vi "Main.vi"(4 "출력 클러스터 2":T1, 5 "RowHdrs":string[](array[string]), 6 "Internal Control":string[][](table)=[["H01", "SYBR", "beta-Actin", "Unkn", "Fl1", "22.22", ""], ["H02", "SYBR", "beta-Actin", "Unkn", "Fl1", "22.27", ""], ["H03", "SYBR", "beta-Actin", "Unkn", "Fl2", "22.94", ""], ["H04", "SYBR", "beta-Actin", "Unkn", "Fl2", "22.82", ""], ["H05", "SYBR", "beta-Actin", "Unkn", "Fl3", "23.04", ""], ["H06", "SYBR", "beta-Actin", "Unkn", "Fl3", "22.72", ""], ["H07", "SYBR", "beta-Actin", "Unkn", "Pfl1", "22.09", ""], ["H08", "SYBR", "beta-Actin", "Unkn", "Pfl1", "22.09", ""], ["H09", "SYBR", "beta-Actin", "Unkn", "Pfl2", "21.57", ""], ["H10", "SYBR", "beta-Actin", "Unkn", "Pfl2", "21.16", ""], ["H11", "SYBR", "beta-Actin", "Unkn", "Pfl3", "21.80", ""], ["H12", "SYBR", "beta-Actin", "Unkn", "Pfl3", "21.93", ""]], 7 "Target Gene":string[][][](array[string])) -> (0 "Result":string[][](table), 1 "Plot data":cluster{i32[], dbl[]}[][](array[cluster]), 3 "Bar (or symbol) plot":picture[][](array[picture]))   [LabVIEW 2015]
uses:
  <vilib>/Analysis/baseanly.llb/Mean (DBL).vi
  <vilib>/Analysis/NI_AALBase.lvlib
panel:
  out "P-value":dbl[](array[numeric])
  out "Report format":string[][](table)
  out "Out":string[](array[string])
  out "Internal Control_Mean":string[](array[string])
  out "Internal Control_Data":string[](array[string])
  out "Gene List":string[](array[string])
  out "Target_Data":string[][](array[string])
  out "2^(-ddCt)":dbl[][](array[numeric])
  out "ddCt":dbl[][](array[numeric])
  out "AVG_dCt_Ctrl":dbl[](array[numeric])
  out "2^(-dCt)":dbl[][](array[numeric])
  out "dCt":dbl[][](array[numeric])
  out "Result Block":string[][][](array[string])
  out "RowHdrs":string[](array[string])
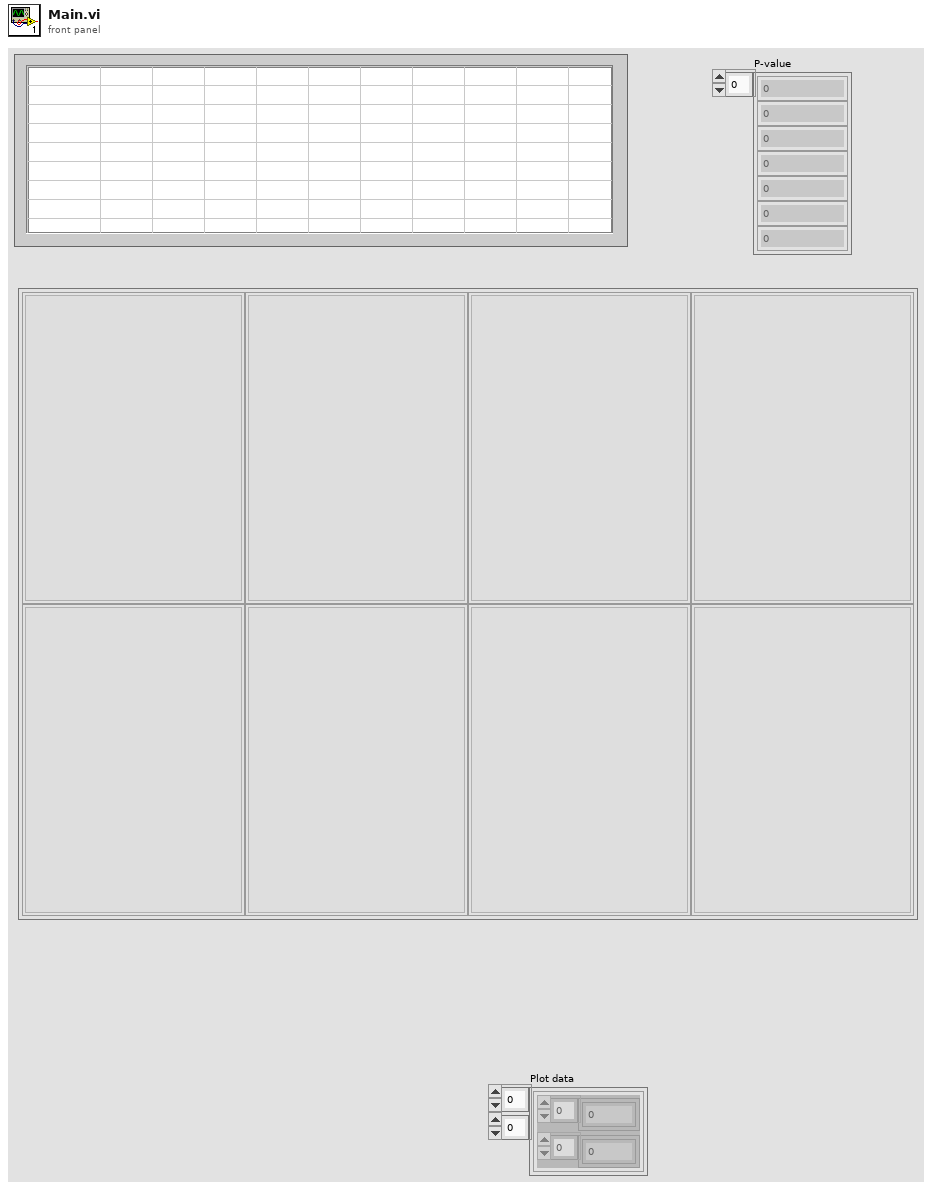
[diagram p1: front panel]
types:
  T1 = cluster{"Group #":dbl, "Biological replicate":dbl, "Technical replicate":dbl}
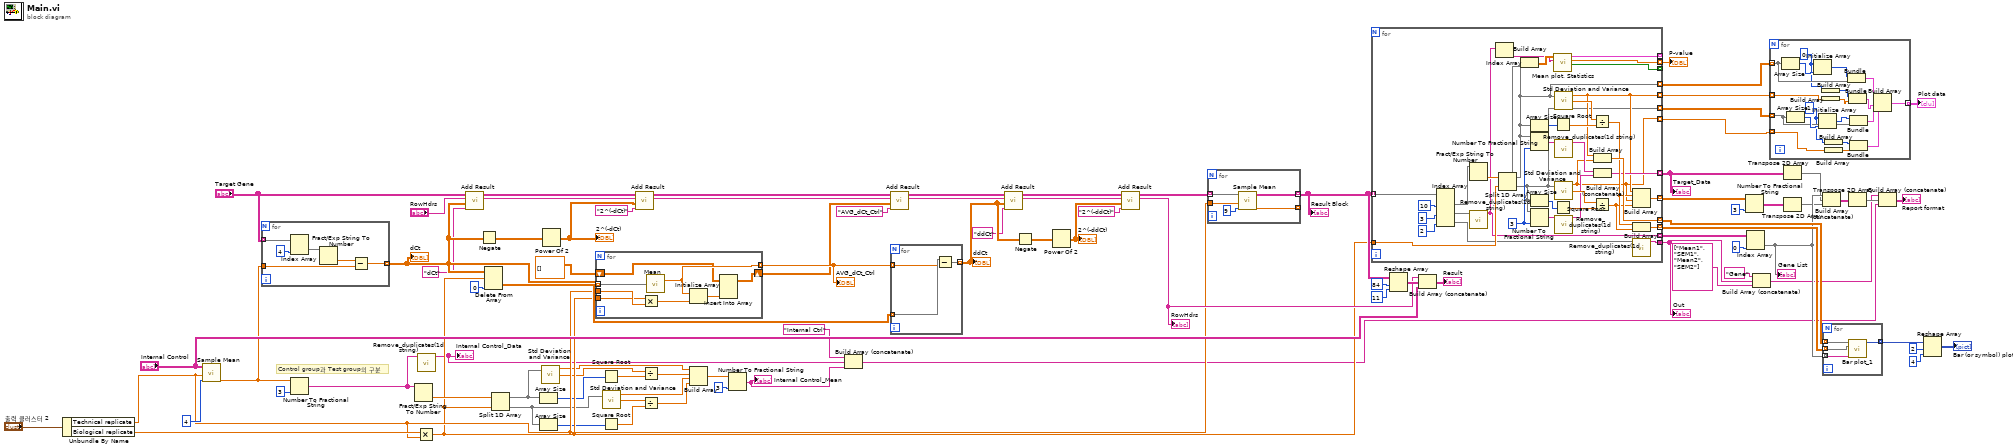
[diagram p0: block diagram]
diagram:
  # "Control group과 Test group의 구분"
  n1 = Unbundle By Name("출력 클러스터 2") -> ("Technical replicate"=w46:dbl, "Biological replicate"=w47:dbl)
  n2 = call "Sample Mean.vi"("Select Data"=4 ("비활성화된 인덱스 (열)"), "Technical replicate"=w46, "Input"="Internal Control") -> ("Sample Average"=w40:dbl[])  [unwired: 7 in, 1 out]
  n3 = for {
    tunnel: "Target Gene" -> [w95] mode=indexing
    tunnel: w40 -> [w91]
    tunnel: [w90] -> w81 mode=indexing
    n4 = Index Array(array=w95, index (col)=4 ("비활성화된 인덱스 (열)")) -> (element=w93:string[])  [unwired: 1 in]
    n5 = Fract/Exp String To Number(string=w93) -> (number=w92:dbl[])  [unwired: 3 in, 1 out]
    n6 = Subtract(x=w92, y=w91) -> (x-y=w90:dbl[])
  }
  "dCt" <- w81
  n7 = Number To Fractional String(number=w40, precision (6)=i16 3 ("정밀도(6)")) -> (F-format string=w38:string[])  [unwired: 2 in]
  n8 = Fract/Exp String To Number(string=w38) -> (number=w39:dbl[])  [unwired: 3 in, 1 out]
  n9 = call <userlib>:"Remove_duplicates(1d string).vi"("In"=w38) -> ("Out"=w9:string[])  [unwired: 10 in]
  "Internal Control_Data" <- w9
  n10 = Multiply(x=w47, y=w46) -> (x*y=w37:dbl)
  n11 = call "Add Result.vi"("Header"="dCt", "dCt"=w81, "RowHdrs Input"="RowHdrs", "Input"="Target Gene") -> ("RowHdrs Output"=w78:string[], "Output"=w79:string[][][])  [unwired: 6 in]
  n12 = Negate(x=w81) -> (-x=w89:dbl[][])
  n13 = Delete From Array(array=w81, length=w37, index (col)=0 ("비활성화된 인덱스 (열)")) -> (deleted portion=w87:dbl[][])  [unwired: 1 in, 1 out]
  n14 = Split 1D Array(array=w39, index=w37) -> (first subarray=w33:dbl[], second subarray=w29:dbl[])
  n15 = Array Size(array=w33) -> (size(s)=w34:i32)
  n16 = Array Size(array=w29) -> (size(s)=w32:i32)
  n17 = call <vilib>:"Std Deviation and Variance.vi"("X"=w33) -> ("mean"=w28:dbl, "standard deviation"=w35:dbl)  [unwired: 1 in, 1 out]
  n18 = Power Of 2(x=w89) -> (2^x=w77:dbl[][])
  "2^(-dCt)" <- w77
  n19 = for {
    tunnel: w87 -> [w103] mode=indexing
    tunnel: [w102] -> w86 mode=indexing
    shift-right: [w99] -> w59
    shift-left: dbl[][] [] -> [w101]
    tunnel: w37 -> [w97]
    tunnel: w46 -> [w98]
    n20 = Multiply(x=w97, y=w98) -> (x*y=w96:dbl)
    n21 = call-poly <vilib>:"Mean.vi"("X"=w103) -> ("mean"=w102:dbl)  [unwired: 1 out]
    n22 = Initialize Array(w102, w96) -> (w100:dbl[])
    n23 = Insert Into Array(array=w101, new element=w100) -> (w99:dbl[][])  [unwired: 2 in]
  }
  "AVG_dCt_Ctrl" <- w86
  n24 = Square Root(x=w34) -> (sqrt(x)=w36:dbl)
  n25 = Square Root(x=w32) -> (sqrt(x)=w30:dbl)
  n26 = call <vilib>:"Std Deviation and Variance.vi"("X"=w29) -> ("mean"=w26:dbl, "standard deviation"=w31:dbl)  [unwired: 1 in, 1 out]
  n27 = call "Add Result.vi"("Header"="2^(-dCt)", "dCt"=w77, "RowHdrs Input"=w78, "Input"=w79) -> ("RowHdrs Output"=w64:string[], "Output"=w63:string[][][])  [unwired: 6 in]
  n28 = Divide(x=w35, y=w36) -> (x/y=w27:dbl)
  n29 = Divide(x=w31, y=w30) -> (x/y=w25:dbl)
  n30 = Build Array(w28, w27, w26, w25) -> (w24:dbl[])
  n31 = Number To Fractional String(number=w24, precision (6)=i16 3 ("정밀도(6)")) -> (F-format string=w8:string[])  [unwired: 2 in]
  "Internal Control_Mean" <- w8
  n32 = Build Array (concatenate)("Internal Ctrl", w9, w8) -> (w7:string[])
  n33 = call "Add Result.vi"("Header"="AVG_dCt_Ctrl", "dCt"=w59, "RowHdrs Input"=w64, "Input"=w63) -> ("RowHdrs Output"=w61:string[], "Output"=w62:string[][][])  [unwired: 6 in]
  n34 = for {
    tunnel: w81 -> [w106] mode=indexing
    tunnel: w86 -> [w105] mode=indexing
    tunnel: [w104] -> w75 mode=indexing
    n35 = Subtract(x=w106, y=w105) -> (x-y=w104:dbl[])
  }
  "ddCt" <- w75
  n36 = call "Add Result.vi"("Header"="ddCt", "dCt"=w75, "RowHdrs Input"=w61, "Input"=w62) -> ("RowHdrs Output"=w73:string[], "Output"=w58:string[][][])  [unwired: 6 in]
  n37 = Negate(x=w75) -> (-x=w85:dbl[][])
  n38 = Power Of 2(x=w85) -> (2^x=w72:dbl[][])
  "2^(-ddCt)" <- w72
  n39 = call "Add Result.vi"("Header"="2^(-ddCt)", "dCt"=w72, "RowHdrs Input"=w73, "Input"=w58) -> ("RowHdrs Output"=w66:string[], "Output"=w57:string[][][])  [unwired: 6 in]
  "RowHdrs" <- w66
  n40 = for {
    tunnel: w57 -> [w111] mode=indexing
    tunnel: [w109] -> w56 mode=indexing
    tunnel: [w108] -> _ mode=indexing
    tunnel: w46 -> [w107]
    n41 = call "Sample Mean.vi"("Select Data"=9, "Technical replicate"=w107, "Input"=w111) -> ("Sample Average"=w108:dbl[], "Output"=w109:string[][])  [unwired: 7 in]
  }
  "Result Block" <- w56
  n42 = for {
    tunnel: w56 -> [w148] mode=indexing
    tunnel: [w138] -> w51 mode=indexing
    tunnel: [w137] -> w50 mode=indexing
    tunnel: w37 -> [w136]
    tunnel: [w133] -> w45 mode=indexing
    tunnel: [w128] -> w21 mode=indexing
    tunnel: [w120] -> w43 mode=indexing
    tunnel: [w122] -> w17
    tunnel: [w118] -> _ mode=indexing
    tunnel: [w117] -> w6 mode=indexing
    tunnel: [w116] -> _ mode=indexing
    tunnel: [w115] -> w5 mode=indexing
    tunnel: [w114] -> w3 mode=indexing
    tunnel: [w113] -> w4 mode=indexing
    tunnel: [w112] -> w2 mode=indexing
    w127 = i16 3 ("정밀도(6)")
    n43 = Index Array(array=w148, index (col) #1=10 ("비활성화된 인덱스 (열)"), index (col) #2=3 ("인덱스 (열)"), index (col) #3=2 ("인덱스 (열)")) -> (element #1=w146:string[], element #2=w125:string[], element #3=w123:string[])  [unwired: 3 in]
    n44 = Fract/Exp String To Number(string=w146) -> (number=w145:dbl[])  [unwired: 3 in, 1 out]
    n45 = call <userlib>:"Remove_duplicates(1d string).vi"("In"=w125) -> ("Out"=w120:string[])  [unwired: 10 in]
    n46 = Index Array(array=w120) -> (element=w119:string)  [unwired: 1 in]
    n47 = Split 1D Array(array=w145, index=w136) -> (first subarray=w115:dbl[], second subarray=w113:dbl[])
    n48 = Build Array(w115, w113) -> (w121:dbl[][])
    n49 = Array Size(array=w115) -> (size(s)=w143:i32)
    n50 = Number To Fractional String(number=w115, precision (6)=w127) -> (F-format string=w132:string[])  [unwired: 2 in]
    n51 = Array Size(array=w113) -> (size(s)=w144:i32)
    n52 = Number To Fractional String(number=w113, precision (6)=w127) -> (F-format string=w131:string[])  [unwired: 2 in]
    n53 = call "Mean plot, Statistics.vi"("Gene Name"=w119, "배열"=w121) -> ("Reject null hypothesis"=w116:bool, "P-value"=w117:dbl, "Plot"=w118:cluster{i32[], "배열":dbl[]}[])  [unwired: 3 in]
    n54 = Square Root(x=w143) -> (sqrt(x)=w141:dbl)
    n55 = Square Root(x=w144) -> (sqrt(x)=w139:dbl)
    n56 = call <vilib>:"Std Deviation and Variance.vi"("X"=w115) -> ("mean"=w114:dbl, "standard deviation"=w142:dbl)  [unwired: 1 in, 1 out]
    n57 = call <userlib>:"Remove_duplicates(1d string).vi"("In"=w132) -> ("Out"=w130:string[])  [unwired: 10 in]
    n58 = call <vilib>:"Std Deviation and Variance.vi"("X"=w113) -> ("mean"=w112:dbl, "standard deviation"=w140:dbl)  [unwired: 1 in, 1 out]
    n59 = call <userlib>:"Remove_duplicates(1d string).vi"("In"=w131) -> ("Out"=w129:string[])  [unwired: 10 in]
    n60 = Divide(x=w142, y=w141) -> (x/y=w135:dbl)
    n61 = Divide(x=w140, y=w139) -> (x/y=w134:dbl)
    n62 = Build Array(w114, w112) -> (w138:dbl[])
    n63 = Build Array (concatenate)(w130, w129) -> (w128:string[])
    n64 = Build Array(w114, w135, w112, w134) -> (w133:dbl[])
    n65 = Build Array(w135, w134) -> (w137:dbl[])
    n66 = call <userlib>:"Remove_duplicates(1d string).vi"("In"=w123) -> ("Out"=w122:string[])  [unwired: 10 in]
  }
  "Target_Data" <- w21
  "Out" <- w17
  "P-value" <- w6
  n67 = Reshape Array(w56, 84 ("차원 크기"), 11 ("차원 크기")) -> (w68:string[][])
  n68 = Build Array (concatenate)(w66, w68, "Internal Control") -> (→"Result":string[][])
  n69 = Number To Fractional String(number=w45, precision (6)=i16 3 ("정밀도(6)")) -> (F-format string=w13:string[][])  [unwired: 2 in]
  n70 = Index Array(array=w43, index (col)=0 ("비활성화된 인덱스 (열)")) -> (element=w22:string[])  [unwired: 1 in]
  "Gene List" <- w22
  n71 = Build Array (concatenate)("Gene", w17, string[] ["Mean1", "SEM1", "Mean2", "SEM2"] ("원소")) -> (w15:string[])
  n72 = for {
    tunnel: [w149] -> w1 mode=indexing
    tunnel: w5 -> [w161] mode=indexing
    tunnel: w4 -> [w160] mode=indexing
    tunnel: w3 -> [w158] mode=indexing
    tunnel: w2 -> [w152] mode=indexing
    w153 = 1 ("원소")
    w159 = 0 ("원소")
    n73 = Array Size(array=w161) -> (size(s)=w167:i32)
    n74 = Array Size(array=w160) -> (size(s)=w166:i32)
    n75 = Initialize Array(w159, w167) -> (w165:i32[])
    n76 = Initialize Array(w153, w166) -> (w164:i32[])
    n77 = Build Array(w159) -> (w156:i32[])
    n78 = Build Array(w158) -> (w157:dbl[])
    n79 = Build Array(w153) -> (w155:i32[])
    n80 = Build Array(w152) -> (w154:dbl[])
    n81 = Bundle(w165, w161) -> (w163:cluster{i32[], dbl[]})  [unwired: 1 in]
    n82 = Bundle(w156, w157) -> (w150:cluster{i32[], dbl[]})  [unwired: 1 in]
    n83 = Bundle(w155, w154) -> (w151:cluster{i32[], dbl[]})  [unwired: 1 in]
    n84 = Bundle(w164, w160) -> (w162:cluster{i32[], dbl[]})  [unwired: 1 in]
    n85 = Build Array(w163, w162, w150, w151) -> (w149:cluster{i32[], dbl[]}[])
  }
  "Plot data" <- w1
  n86 = Transpose 2D Array(2D array=w21) -> (transposed array=w20:string[][])
  n87 = Transpose 2D Array(2D array=w13) -> (transposed array=w12:string[][])
  n88 = Build Array (concatenate)(w22, w20, w12) -> (w19:string[][])
  n89 = for {
    tunnel: w51 -> [w171] mode=indexing
    tunnel: w50 -> [w170] mode=indexing
    tunnel: [w169] -> w52 mode=indexing
    tunnel: w22 -> [w168] mode=indexing
    n90 = call "Bar plot_1.vi"("Gene Name"=w168, "SEM"=w170, "MEAN"=w171) -> ("2^(-ddCT)"=w169:picture)  [unwired: 4 in]
  }
  n91 = Transpose 2D Array(2D array=w19) -> (transposed array=w18:string[][])
  n92 = Build Array (concatenate)(w15, w18, w7) -> (→"Report format":string[][])
  n93 = Reshape Array(w52, 2 ("차원 크기"), 4 ("차원 크기")) -> (→"Bar (or symbol) plot":picture[][])
